vi "NestedActorLaunched.vi"(8 "error in (no error)":errorcluster, 10 "NestedActorName":T1, 11 "MFActor in":refnum<class "MFActor.lvclass">) -> (0 "error out":errorcluster, 3 "MFActor out":refnum<class "MFActor.lvclass">)   [LabVIEW 2024, in "MFActor.lvlib" / "MFActor.lvclass"]
uses:
  MFActor.lvclass
  NestedActorName.ctl
  MFActor.lvclass/MFActor.ctl
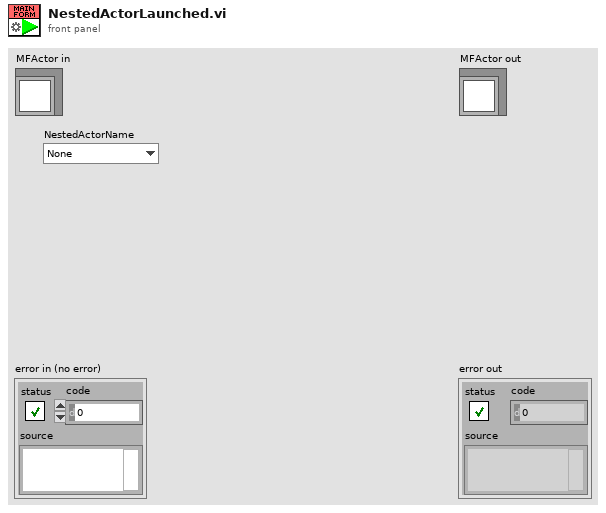
[diagram p1: front panel]
types:
  T1 = typedef "NestedActorName.ctl" = enum16{"None", "4503#0", "4503#1", "AIO#0", "AIO#1", "DIO", "PID", "TCPIP", "TestAngle", "TestFixPt", "TestMultiPt", "TestSinWave", "PW3390", "ADAM4118"}
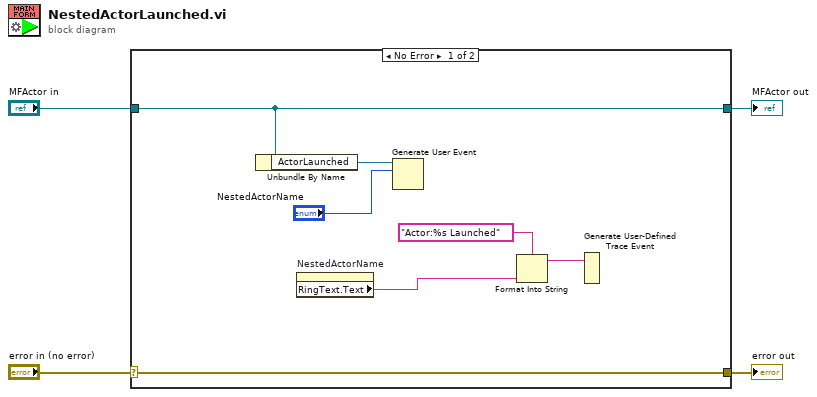
[diagram p0: block diagram]
diagram:
  n1 = case shown="No Error" "error in (no error)" {
    selector: "error in (no error)" -> [w11 w13]
    tunnel: [w11 w13] -> w3
    tunnel: [w10 w12] -> w1
    tunnel: "MFActor in" -> [w10 w12]
    frame No Error {
      n2 = Unbundle By Name(w10) -> ("ActorLaunched"=w9:refnum<user-event>)
      n3 = property on="NestedActorName" class="Enum (strict)"() -> ("RingText.Text"=w5:string)  [unwired: 2 in, 2 out]
      n4 = Generate User Event(user event=w9, event data cluster="NestedActorName") -> ()  [unwired: 2 in, 2 out]
      n5 = Format Into String(format string="Actor:%s Launched" ("trace string"), w5) -> (resulting string=w6:string)  [unwired: 2 in, 1 out]
      n6 = Generate User-Defined Trace Event(2:w6) -> ()  [unwired: 1 in]
    }
    frame Error {
    }
  }
  "error out" <- w3
  "MFActor out" <- w1
